vi "AutoCameraBased.vi"(8 "Int Parameter":dbl, 10 "Letter Code":string, 11 "Drive Speed":dbl) -> ()   [LabVIEW 2016]
uses:
  Robot Global Data.vi
  <vilib>/Rock Robotics/WPI/Utilities/WPI_GetSetVariantRefNum.vi
  <vilib>/Rock Robotics/WPI/RobotDrive/WPI_RobotDriveMecanumDrive_Cartesian.vi
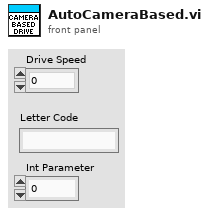
[diagram p1: front panel]
types:
  T1 = typedef "WPI_RobotDriveDevRef.ctl" = cluster{"DevStatus":errorcluster, "Motors[]":T2[], "Square Inputs":bool, "Max Output":dbl}
  T2 = typedef "WPI_MotorControlDeviceRef.ctl" = cluster{"DeviceStatus":errorcluster, "Type":T3, "PWM":cluster{"PWM Channel":T4, "DeadBand":T5}, "CAN":cluster{"Device Number":u8, "SetOutput VI Ref":variant, "GetOutput VI Ref":variant, "Enable VI Ref":variant, "Disable VI Ref":variant, "Data":variant}, "Invert":bool}
  T3 = typedef "WPI_MotorControlType.ctl" = enum16{"PWM", "CAN"}
  T4 = typedef "FPGA_DIOPWMChannel.ctl" = enum8{"PWM 0", "PWM 1", "PWM 2", "PWM 3", "PWM 4", "PWM 5", "PWM 6", "PWM 7", "PWM 8", "PWM 9", "PWM MXP 0", "PWM MXP 1", "PWM MXP 2", "PWM MXP 3", "PWM MXP 4", "PWM MXP 5", "PWM MXP 6", "PWM MXP 7", "PWM MXP 8", "PWM MXP 9", "Invalid"}
  T5 = typedef "WPI_PWMDeadband.ctl" = cluster{"Name":string, "maxPositivePwm":i32, "minPositivePwm":i32, "centerPwm":i32, "maxNegativePwm":i32, "minNegativePwm":i32, "angularRange":u16}
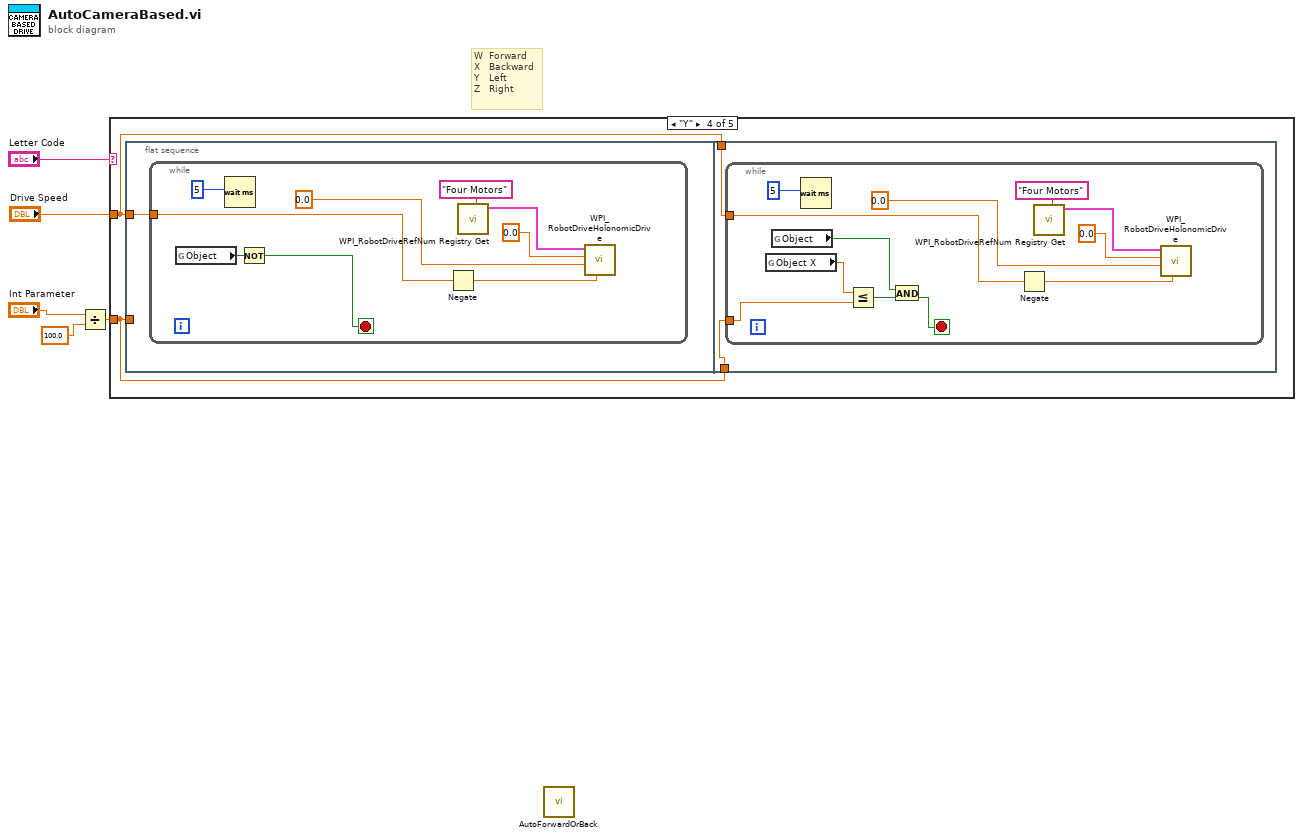
[diagram p0: block diagram]
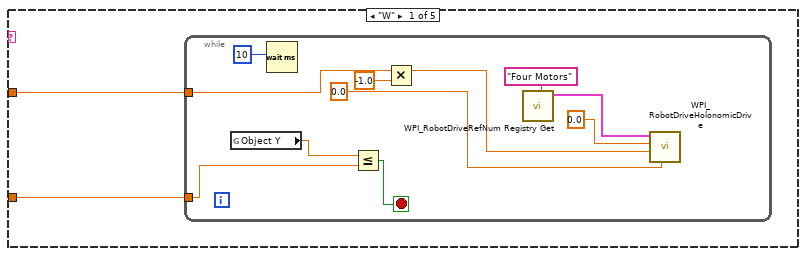
[diagram p2: hidden frame]
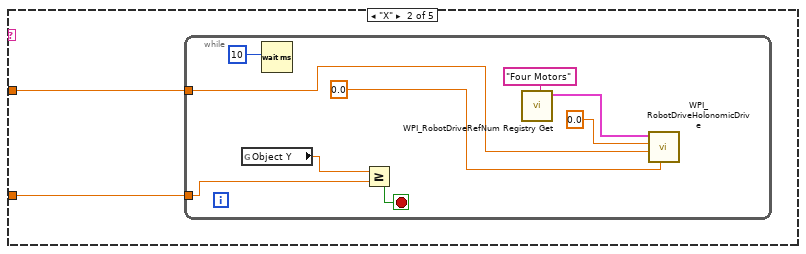
[diagram p3: hidden frame]
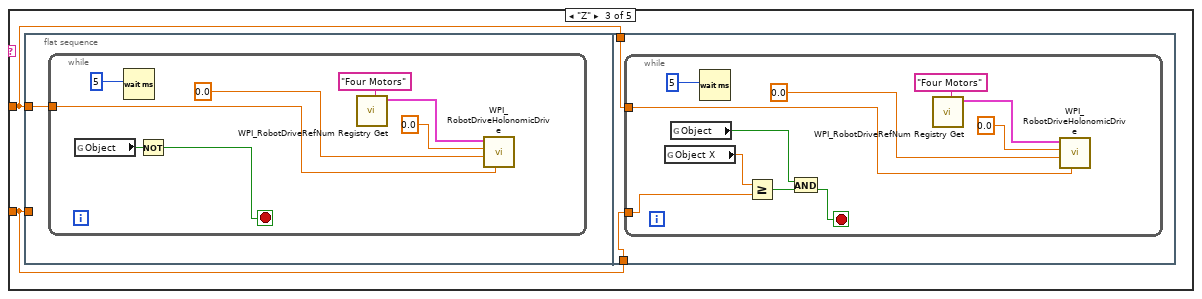
[diagram p4: hidden frame]
diagram:
  # "W  Forward\nX   Backward\nY   Left\nZ   Right"
  n1 = Divide(x="Int Parameter", y=100.0) -> (x/y=w1:dbl)
  n2 = case shown="\"Y\"" "Letter Code" {
    tunnel: "Drive Speed" -> [w7 w20 w30 w54 _]
    tunnel: w1 -> [w6 w19 w31 w55 _]
    frame "W" {
      n3 = while {
        tunnel: w7 -> [w13]
        tunnel: w6 -> [w10]
        stop <- w11 stop-if-true
        n4 = global read "Robot Global Data.vi" "Object Y"() -> (w12:dbl)
        n5 = Wait (ms)(milliseconds to wait=10) -> ()  [unwired: 1 out]
        n6 = Less Or Equal?(x=w12, y=w10) -> (x <= y?=w11:bool)
        n7 = Multiply(x=w13, y=-1.0) -> (x*y=w9:dbl)
        n8 = call <vilib>:"WPI_RobotDriveRefNum Registry Get.vi"("refnum name"="Four Motors") -> ("RobotDriveDevRef"=w17:T1)  [unwired: 9 in, 1 out]
        n9 = call-poly <vilib>:"WPI_RobotDriveHolonomicDrive.vi"("Rotation"=0.0, "Y"=w9, "X"=0.0, "RobotDriveDevRef"=w17) -> ()  [unwired: 5 in, 3 out]
      }
    }
    frame "X" {
      n10 = while {
        tunnel: w20 -> [w24]
        tunnel: w19 -> [w22]
        stop <- w21 stop-if-true
        n11 = global read "Robot Global Data.vi" "Object Y"() -> (w23:dbl)
        n12 = Wait (ms)(milliseconds to wait=10) -> ()  [unwired: 1 out]
        n13 = Greater Or Equal?(x=w23, y=w22) -> (x >= y?=w21:bool)
        n14 = call <vilib>:"WPI_RobotDriveRefNum Registry Get.vi"("refnum name"="Four Motors") -> ("RobotDriveDevRef"=w26:T1)  [unwired: 9 in, 1 out]
        n15 = call-poly <vilib>:"WPI_RobotDriveHolonomicDrive.vi"("Rotation"=0.0, "Y"=w24, "X"=0.0, "RobotDriveDevRef"=w26) -> ()  [unwired: 5 in, 3 out]
      }
    }
    frame "Z" {
      n16 = flat-sequence {
        tunnel: w30 -> [w32]
        tunnel: w31 -> [_]
        tunnel: w31 -> [w42]
        tunnel: w30 -> [w41]
        frame #0 {
          n17 = while {
            tunnel: w32 -> [w36]
            stop <- w33 stop-if-true
            n18 = global read "Robot Global Data.vi" "Object"() -> (w34:bool)
            n19 = Wait (ms)(milliseconds to wait=5) -> ()  [unwired: 1 out]
            n20 = Not(x=w34) -> (.not. x?=w33:bool)
            n21 = call <vilib>:"WPI_RobotDriveRefNum Registry Get.vi"("refnum name"="Four Motors") -> ("RobotDriveDevRef"=w37:T1)  [unwired: 9 in, 1 out]
            n22 = call-poly <vilib>:"WPI_RobotDriveHolonomicDrive.vi"("Rotation"=w36, "Y"=0.0, "X"=0.0, "RobotDriveDevRef"=w37) -> ()  [unwired: 5 in, 3 out]
          }
        }
        frame #1 {
          n23 = while {
            tunnel: w41 -> [w49]
            tunnel: w42 -> [w45]
            stop <- w44 stop-if-true
            n24 = global read "Robot Global Data.vi" "Object X"() -> (w46:dbl)
            n25 = global read "Robot Global Data.vi" "Object"() -> (w43:bool)
            n26 = Wait (ms)(milliseconds to wait=5) -> ()  [unwired: 1 out]
            n27 = Greater Or Equal?(x=w46, y=w45) -> (x >= y?=w47:bool)
            n28 = And(x=w43, y=w47) -> (x .and. y?=w44:bool)
            n29 = call <vilib>:"WPI_RobotDriveRefNum Registry Get.vi"("refnum name"="Four Motors") -> ("RobotDriveDevRef"=w50:T1)  [unwired: 9 in, 1 out]
            n30 = call-poly <vilib>:"WPI_RobotDriveHolonomicDrive.vi"("Rotation"=w49, "Y"=0.0, "X"=0.0, "RobotDriveDevRef"=w50) -> ()  [unwired: 5 in, 3 out]
          }
        }
      }
    }
    frame "Y" {
      n31 = flat-sequence {
        tunnel: w54 -> [w56]
        tunnel: w55 -> [_]
        tunnel: w55 -> [w67]
        tunnel: w54 -> [w66]
        frame #0 {
          n32 = while {
            tunnel: w56 -> [w61]
            stop <- w58 stop-if-true
            n33 = global read "Robot Global Data.vi" "Object"() -> (w59:bool)
            n34 = Wait (ms)(milliseconds to wait=5) -> ()  [unwired: 1 out]
            n35 = Not(x=w59) -> (.not. x?=w58:bool)
            n36 = Negate(x=w61) -> (-x=w57:dbl)
            n37 = call <vilib>:"WPI_RobotDriveRefNum Registry Get.vi"("refnum name"="Four Motors") -> ("RobotDriveDevRef"=w62:T1)  [unwired: 9 in, 1 out]
            n38 = call-poly <vilib>:"WPI_RobotDriveHolonomicDrive.vi"("Rotation"=w57, "Y"=0.0, "X"=0.0, "RobotDriveDevRef"=w62) -> ()  [unwired: 5 in, 3 out]
          }
        }
        frame #1 {
          n39 = while {
            tunnel: w66 -> [w75]
            tunnel: w67 -> [w71]
            stop <- w70 stop-if-true
            n40 = global read "Robot Global Data.vi" "Object X"() -> (w72:dbl)
            n41 = global read "Robot Global Data.vi" "Object"() -> (w69:bool)
            n42 = Wait (ms)(milliseconds to wait=5) -> ()  [unwired: 1 out]
            n43 = Less Or Equal?(x=w72, y=w71) -> (x <= y?=w73:bool)
            n44 = And(x=w69, y=w73) -> (x .and. y?=w70:bool)
            n45 = Negate(x=w75) -> (-x=w68:dbl)
            n46 = call <vilib>:"WPI_RobotDriveRefNum Registry Get.vi"("refnum name"="Four Motors") -> ("RobotDriveDevRef"=w76:T1)  [unwired: 9 in, 1 out]
            n47 = call-poly <vilib>:"WPI_RobotDriveHolonomicDrive.vi"("Rotation"=w68, "Y"=0.0, "X"=0.0, "RobotDriveDevRef"=w76) -> ()  [unwired: 5 in, 3 out]
          }
        }
      }
    }
    frame Default {
    }
  }
  n48 = call "AutoForwardOrBack.vi"() -> ()  [unwired: 12 in]
